vi "PH_Trendviewer_Powermeter.set Start.vi"(0 "i ref in":refnum<vi>, 1 "Start":bool, 5 "error in (no error)":errorcluster) -> (14 "i ref out":refnum<vi>, 19 "error out":errorcluster)   [LabVIEW 2014, in "PH_Trendviewer_Powermeter.lvlib"]
doc: "This VI sets attributes and some GUI elements. It contains the get data to modify / set modified data -vis, handle with care!"
uses:
  PH_Trendviewer_Powermeter.lvlib
  PH_Common/PH_Common.lvlib
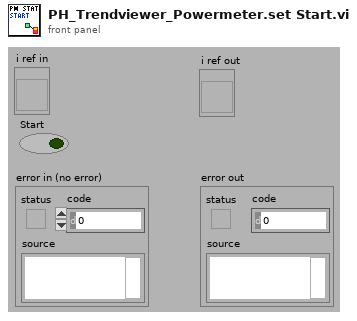
[diagram p1: front panel]
types:
  T1 = typedef "PH_Trendviewer_Powermeter.lvlib/PH_Trendviewer_Powermeter.i attribute.ctl" = cluster{"GUI Refs ":cluster{"Status":refnum<vi>, "Result Graph":refnum<vi>, "Mean Data":refnum<vi>, "Std Dev Data":refnum<vi>, "Dummy Mean":refnum<vi>, "Dummy Std Dev":refnum<vi>, "Export Data":refnum<vi>, "Stat or Trend":refnum<vi>, "Delete":refnum<vi>, "Powermeter":refnum<vi>, "Start":refnum<vi>}, "Powermeter":string, "Stat or Trend":bool, "Start":bool, "Data":cluster{"Time Stamp":timestamp, "Energy [J]":dbl}[], "Datasets strored":i32, "Dataarray Size":i32}
  T2 = enum8{"Enabled", "Disabled", "Disabled and Grayed Out"}
  T3 = cluster{"Time Stamp":timestamp, "Energy [J]":dbl}[]
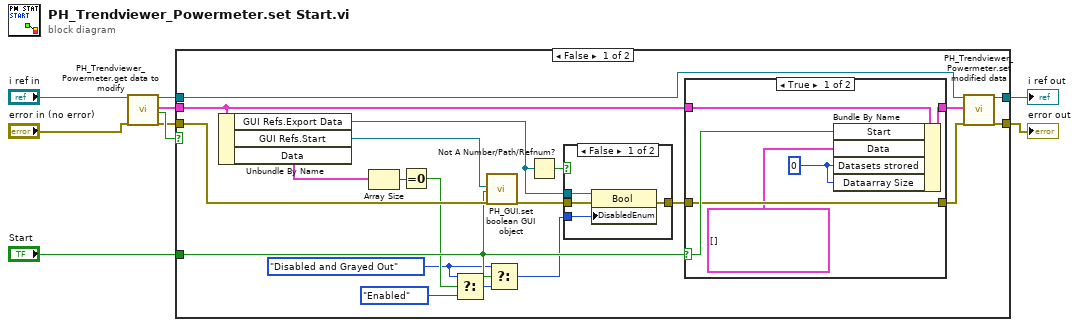
[diagram p0: block diagram]
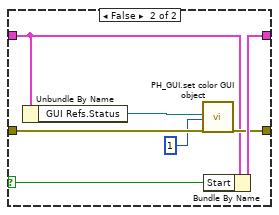
[diagram p3: hidden frame]
diagram:
  n1 = call "PH_Trendviewer_Powermeter.get data to modify.vi"("i ref in"="i ref in", "error in (no error)"="error in (no error)") -> ("i ref out"=w4:refnum<vi>, "i attribute"=w8:T1, "timed out"=w7:bool, "error out"=w3:errorcluster)  [unwired: 14 in]
  n2 = case shown="False" w7 {
    tunnel: w3 -> [w24 w48]
    tunnel: w4 -> [w21 w49]
    tunnel: [w29 w49] -> w5
    tunnel: [w28 w48] -> w6
    tunnel: w8 -> [w26 _]
    tunnel: "Start" -> [w17 _]
    frame False {
      w12 = T2."Disabled and Grayed Out" ("t")
      n3 = Unbundle By Name(w26) -> ("GUI Refs.Export Data"=w18:refnum<vi>, "GUI Refs.Start"=w25:refnum<vi>, "Data"=w15:T3)
      n4 = Array Size(array=w15) -> (size(s)=w14:i32)
      n5 = Equal To 0?(x=w14) -> (x = 0?=w13:bool)
      n6 = Select(t=w12, s=w13, f=T2."Enabled" ("Disabled")) -> (s? t:f=w10:T2)
      n7 = call "PH_GUI.set boolean GUI object.vi"("Boolean Knob GUI Ref"=w25, "Value"=w17, "error in (no error)"=w24) -> ("error out"=w23:errorcluster)  [unwired: 16 in]
      n8 = Select(t=w12, s=w17, f=w10) -> (s? t:f=w16:T2)
      n9 = Not A Number/Path/Refnum?(number/path/refnum=w18) -> (NaN/Path/Refnum?=w19:bool)
      n10 = case shown="False" w19 {
        tunnel: w23 -> [w33 w34]
        tunnel: [w32 w34] -> w20
        tunnel: w18 -> [w31 _]
        tunnel: w16 -> [w30 _]
        frame False {
          n11 = property class="Bool"(reference=w31, error in=w33, "DisabledEnum"=w30) -> (error out=w32:errorcluster)  [unwired: 1 out]
        }
        frame True {
        }
      }
      n12 = case shown="True" w17 {
        selector: w17 -> [w38 w46]
        tunnel: [w40 w47] -> w27
        tunnel: w26 -> [w39 w43]
        tunnel: w20 -> [w37 w45]
        tunnel: [w37 w44] -> w22
        frame True {
          w35 = 0 ("Datasets strored")
          n13 = Bundle By Name(cluster=w39, "Start"=w38, "Data"=T3 [], "Datasets strored"=w35, "Dataarray Size"=w35) -> (w40:T1)
        }
        frame False {
          n14 = Unbundle By Name(w43) -> ("GUI Refs.Status"=w42:refnum<vi>)
          n15 = call "PH_GUI.set color GUI object.vi"("GUI object Ref"=w42, "State"=1, "error in (no error)"=w45) -> ("error out"=w44:errorcluster)  [unwired: 16 in]
          n16 = Bundle By Name(cluster=w43, "Start"=w46) -> (w47:T1)
        }
      }
      n17 = call "PH_Trendviewer_Powermeter.set modified data.vi"("i ref in"=w21, "i attribute"=w27, "error in (no error)"=w22) -> ("i ref out"=w29:refnum<vi>, "error out"=w28:errorcluster)  [unwired: 15 in]
    }
    frame True {
    }
  }
  "error out" <- w6
  "i ref out" <- w5
